vi "MultiStationGasMeter_Rev0.vi"() -> ()   [LabVIEW 2014]
uses:
  <vilib>/DAQmx/read.llb/DAQmx Read (Analog 1D DBL NChan 1Samp).vi
  <vilib>/DAQmx/miscellaneous.llb/DAQmx Fill In Error Info.vi
panel:
  in  "HeatingValueLP 3":dbl=990.0 min=900.0 max=2600.0 step=1.0
  in  "HeatingValueNG 3":dbl=990.0 min=900.0 max=1200.0 step=1.0
  in  "Start ANSI 3":bool
  out "ANSI Average (BTU/hr) 3":dbl format="%#_5g"
  out "30 Second Average (BTU/hr) 3":dbl format="%#_5g"
  out "15 Second Average (BTU/hr) 3":dbl format="%#_5g"
  out "Signal 3":bool
  out "CF/HR 3":dbl format="%#_2g"
  out "HV 3":dbl
  out "Meter ID 3":dbl
  out "Gas 3":string
  out "DisplayChart 3":cluster{"Flow Rate":dbl}(graph)
  out "Flow Rate 3":dbl format="%#_5g"
  in  "HeatingValueLP 2":dbl=990.0 min=900.0 max=2600.0 step=1.0
  in  "Start ANSI 2":bool
  out "ANSI Average (BTU/hr) 2":dbl format="%#_5g"
  out "30 Second Average (BTU/hr) 2":dbl format="%#_5g"
  out "15 Second Average (BTU/hr) 2":dbl format="%#_5g"
  out "Signal 2":bool
  out "CF/HR 2":dbl format="%#_2g"
  out "HV 2":dbl
  in  "HeatingValueNG 2":dbl=990.0 min=900.0 max=1200.0 step=1.0
  out "Meter ID 2":dbl
  out "Gas 2":string
  out "DisplayChart 2":cluster{"Flow Rate":dbl}(graph)
  out "Flow Rate 2":dbl format="%#_5g"
  out "ANSI Placeholder 3":dbl
  out "Start Time ANSI 3":dbl
  out "ANSI Placeholder 2":dbl
  out "Start Time ANSI 2":dbl
  out "Meter 6 Present":bool
  out "Meter 5 Present":bool
  out "Meter 4 Present":bool
  out "Meter 3 Present":bool
  out "Meter 2 Present":bool
  out "Meter 1 Present":bool
  out "Meter Type 6":string
  out "Meter Type 2":string
  out "Meter Type 4":string
  out "Meter Type 5":string
  out "Meter Type 3":string
  out "Meter Type 1":string
  out "Meter 6 Size":dbl
  out "Meter 5 Size":dbl
  out "Meter 4 Size":dbl
  out "Meter 3 Size":dbl
  out "Meter 2 Size":dbl
  out "Meter 1 Size":dbl
  out "ANSI Placeholder":dbl
  out "Start Time ANSI":dbl
  in  "Start ANSI":bool
  out "ANSI Average (BTU/hr)":dbl format="%#_5g"
  out "30 Second Average (BTU/hr)":dbl format="%#_5g"
  out "15 Second Average (BTU/hr)":dbl format="%#_5g"
  out "Reference6":dbl
  out "Reference5":dbl
  out "Reference4":dbl
  out "Reference3":dbl
  out "Reference2":dbl
  out "Reference1":dbl
  out "Time":dbl
  out "Num Record":dbl
  in  "HeatingValueLP":dbl=2450.0 min=2400.0 max=2600.0 step=1.0
  out "Output 6":dbl min=0.0 max=5.0 step=0.01
  out "Output 5":dbl min=0.0 max=5.0 step=0.01
  out "Output 4":dbl min=0.0 max=5.0 step=0.01
  out "Output 3":dbl min=0.0 max=5.0 step=0.01
  out "Output 2":dbl min=0.0 max=5.0 step=0.01
  out "Output 1":dbl min=0.0 max=5.0 step=0.01
  out "Signal":bool
  in  "Record":bool
  out "File Path":path
  out "CF/HR":dbl format="%#_2g"
  out "HV":dbl
  in  "HeatingValueNG":dbl=990.0 min=900.0 max=1200.0 step=1.0
  out "Meter ID":dbl
  out "Gas":string
  out "DisplayChart":cluster{"Flow Rate":dbl}(graph)
  out "Flow Rate":dbl format="%#_5g"
  # "STATION 1"
  # "STATION 2"
  # "STATION 3"
  # "Heating Value"
  # "Heating Value"
  # "Heating Value"
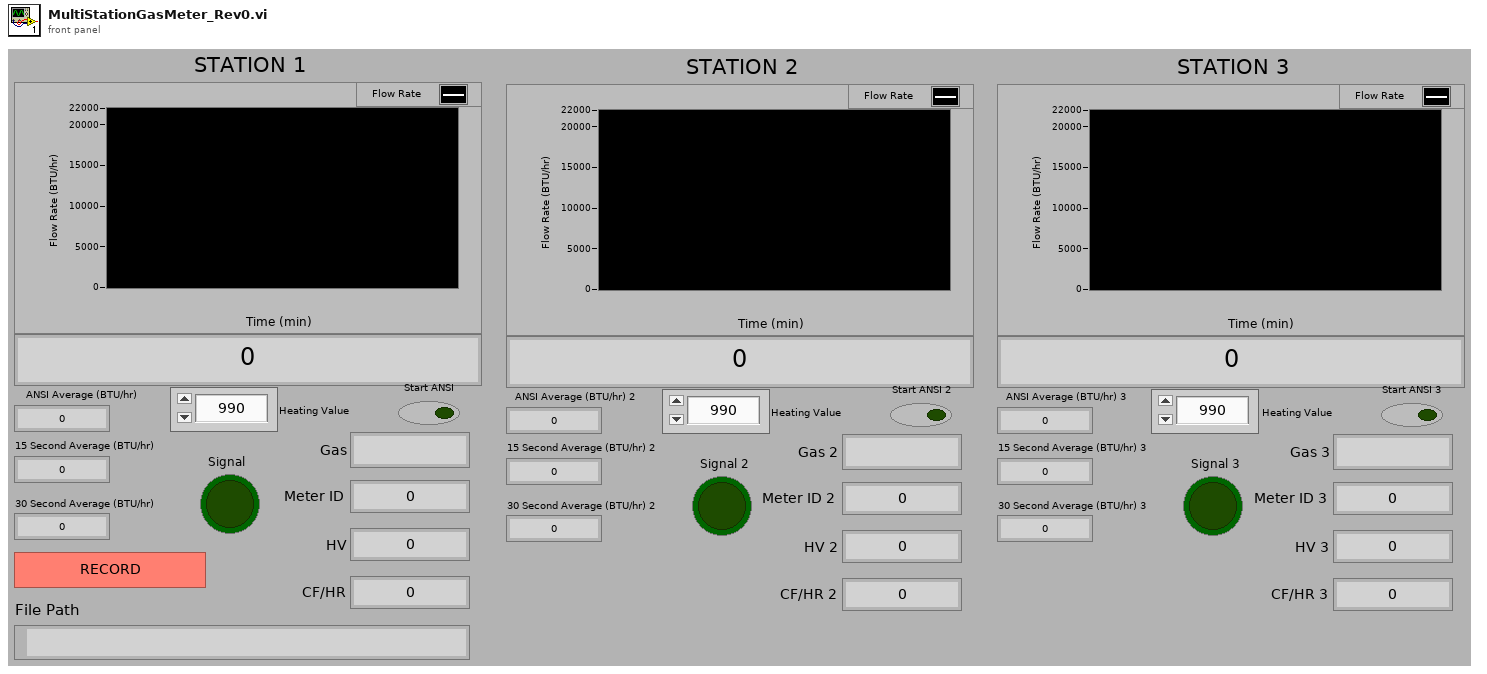
[diagram p1: front panel]
types:
  T1 = enum16{"open", "replace", "create", "open or create", "replace or create", "replace or create with confirmation"}
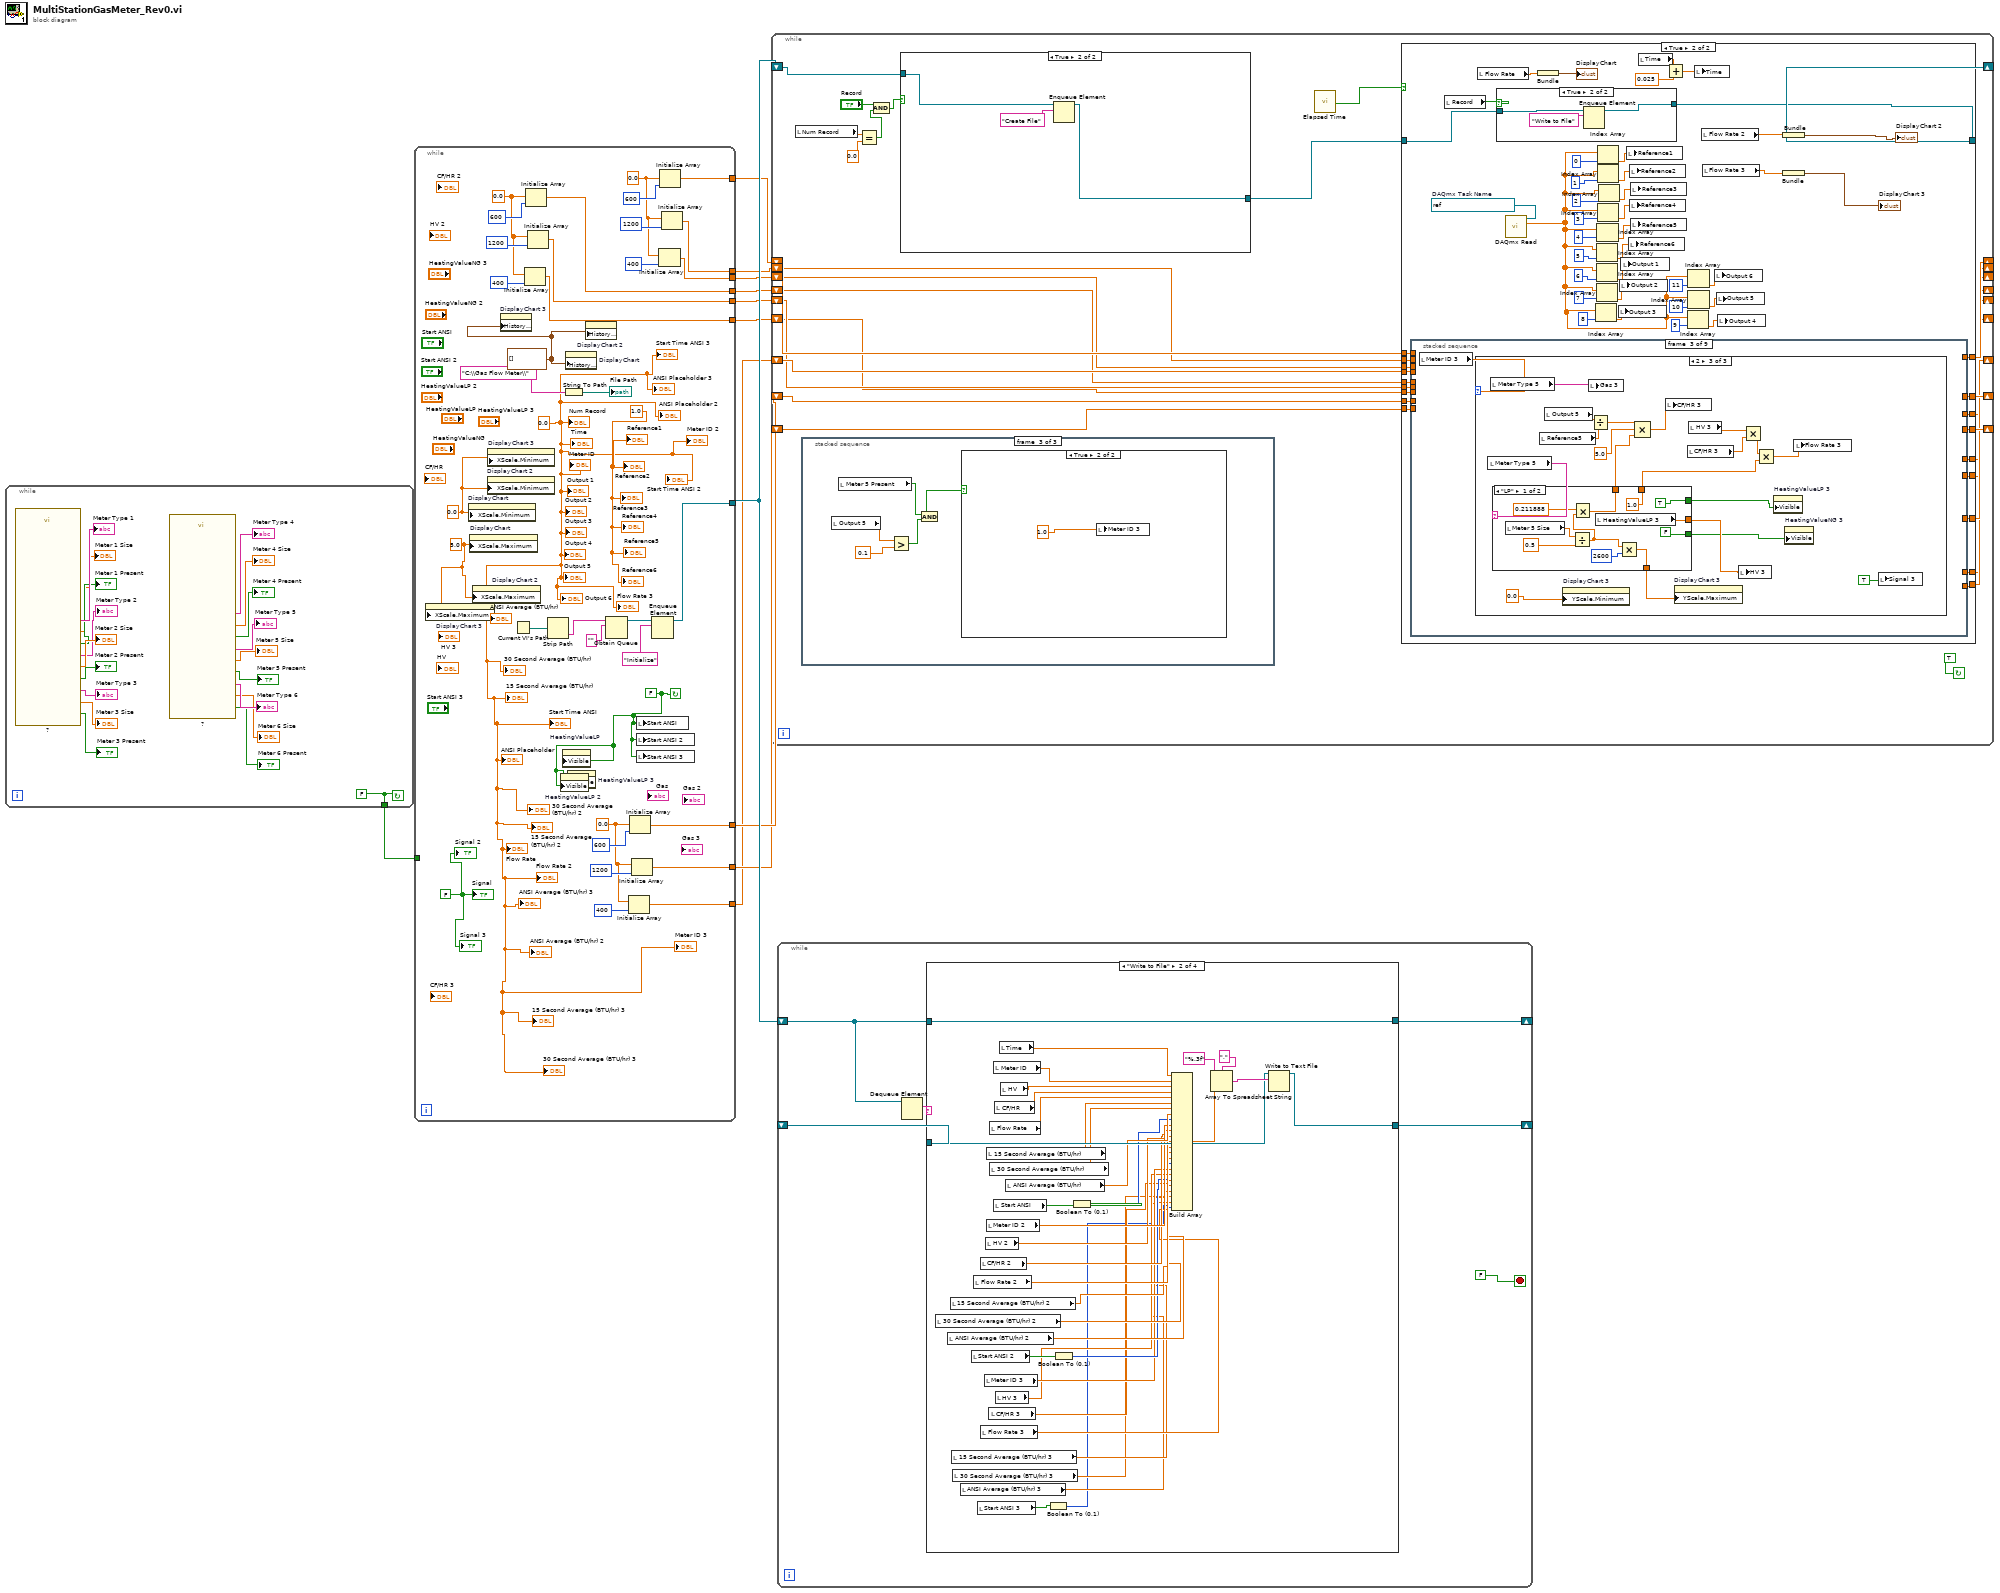
[diagram p0: block diagram]
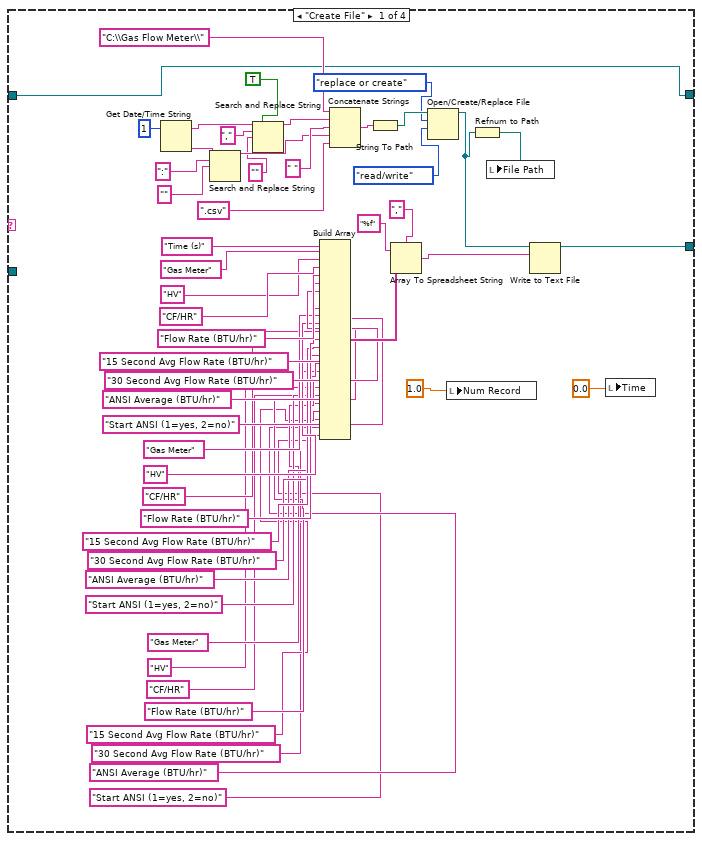
[diagram p2: hidden frame]
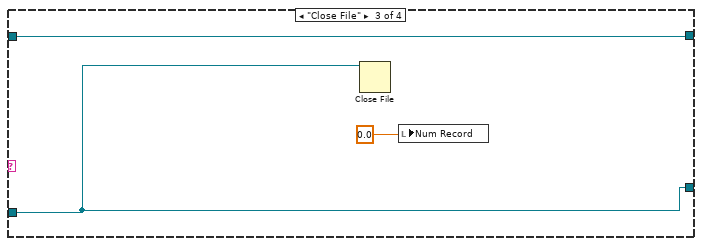
[diagram p3: hidden frame]
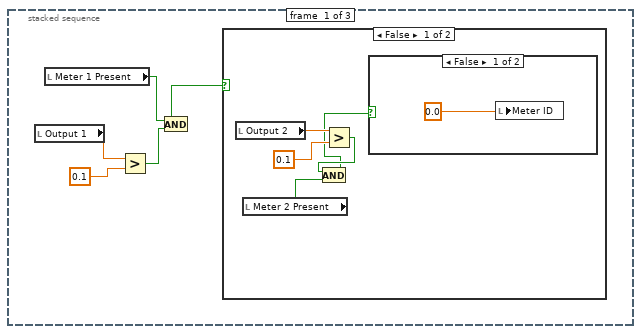
[diagram p5: hidden frame]
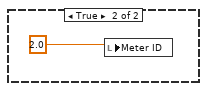
[diagram p6: hidden frame]
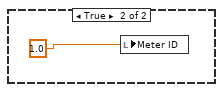
[diagram p7: hidden frame]
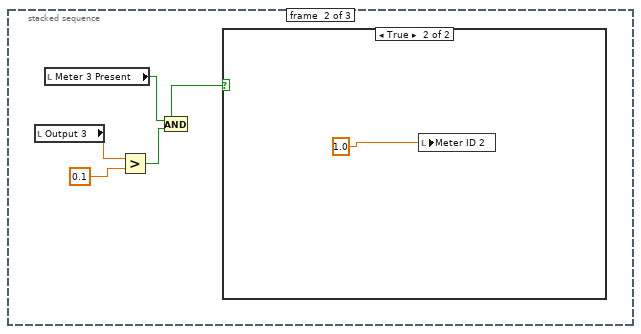
[diagram p8: hidden frame]
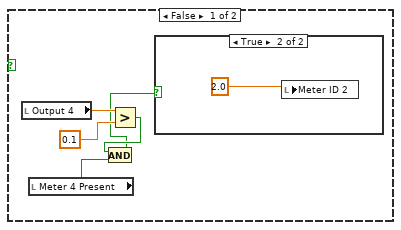
[diagram p9: hidden frame]
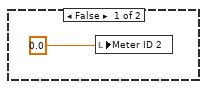
[diagram p10: hidden frame]
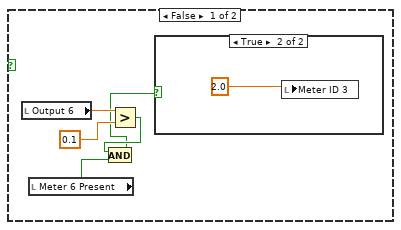
[diagram p11: hidden frame]
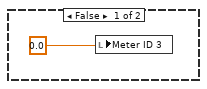
[diagram p12: hidden frame]
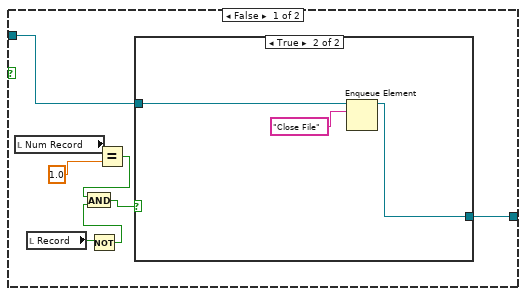
[diagram p13: hidden frame]
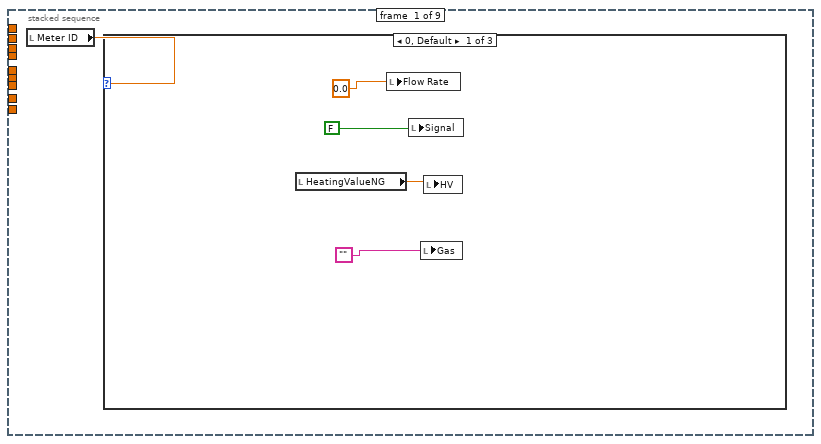
[diagram p16: hidden frame]
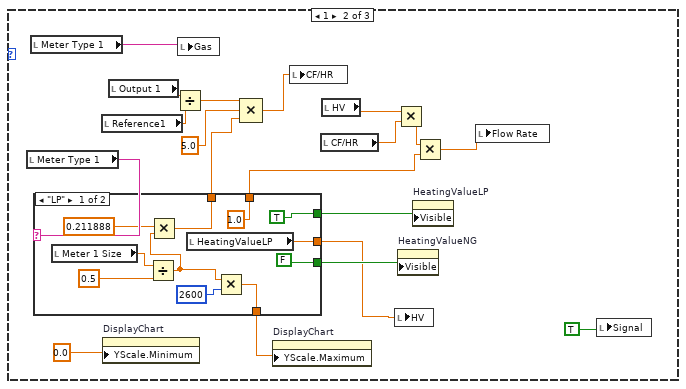
[diagram p17: hidden frame]
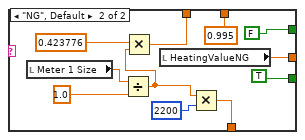
[diagram p18: hidden frame]
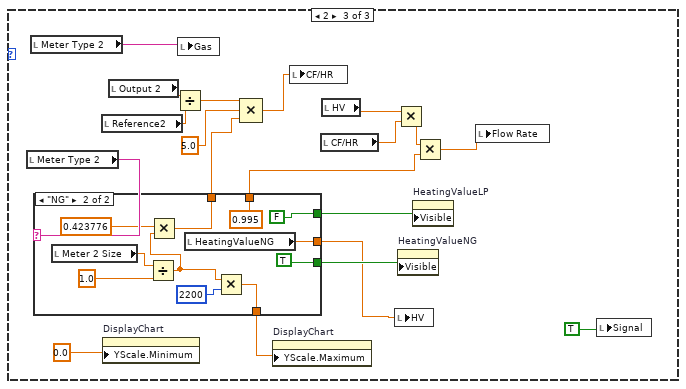
[diagram p19: hidden frame]
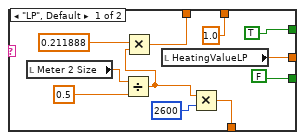
[diagram p20: hidden frame]
diagram:
  n1 = while {
    tunnel: [w29] -> w7
    stop <- w29 continue-if-true
    w29 = FALSE
    n2 = call "?"() -> ("Meter 3 Present?"=→"Meter 3 Present":bool, "Meter Size 3 (SLPM)"=→"Meter 3 Size":dbl, "Meter Type 3 (LP/NG)"=→"Meter Type 3":string, "Meter 2 Present?"=→"Meter 2 Present":bool, "Meter Size 2 (SLPM)"=→"Meter 2 Size":dbl, "Meter Type 2 (LP/NG)"=→"Meter Type 2":string, "Meter 1 Present?"=→"Meter 1 Present":bool, "Meter Size 1 (SLPM)"=→"Meter 1 Size":dbl, "Meter Type 1 (LP/NG)"=→"Meter Type 1":string)  [unwired: 9 in, 2 out]
    n3 = call "?"() -> ("Meter 6 Present?"=→"Meter 6 Present":bool, "Meter Size 6 (SLPM)"=→"Meter 6 Size":dbl, "Meter Type 6 (LP/NG)"=→"Meter Type 6":string, "Meter 5 Present?"=→"Meter 5 Present":bool, "Meter Size 5 (SLPM)"=→"Meter 5 Size":dbl, "Meter Type 5 (LP/NG)"=→"Meter Type 5":string, "Meter 4 Present?"=→"Meter 4 Present":bool, "Meter Size 4 (SLPM)"=→"Meter 4 Size":dbl, "Meter Type 4 (LP/NG)"=→"Meter Type 4":string)  [unwired: 9 in, 2 out]
  }
  n4 = while {
    tunnel: [w60] -> w11
    tunnel: [w56] -> w10
    tunnel: [w55] -> w9
    tunnel: [w52] -> w8
    tunnel: w7 -> [_]
    tunnel: [w47] -> w6
    tunnel: [w46] -> w5
    tunnel: [w45] -> w4
    tunnel: [w40] -> w3
    tunnel: [w39] -> w2
    tunnel: [w38] -> w1
    stop <- w36 continue-if-true
    w42 = 0.0
    w49 = 0.0
    w35 = FALSE
    w54 = 0.0
    w31 = 5.0
    w32 = 0.0
    w59 = 1.0
    w34 = 0.0
    w33 = cluster{"[0]":dbl}[] []
    w36 = FALSE
    n5 = property on="DisplayChart 3" class="WFChart (strict)"("XScale.Maximum"=w31) -> ()  [unwired: 2 in, 2 out]
    n6 = property on="DisplayChart" class="WFChart (strict)"("XScale.Minimum"=w32) -> ()  [unwired: 2 in, 2 out]
    n7 = property on="DisplayChart" class="WFChart (strict)"("XScale.Maximum"=w31) -> ()  [unwired: 2 in, 2 out]
    n8 = property on="DisplayChart 2" class="WFChart (strict)"("XScale.Maximum"=w31) -> ()  [unwired: 2 in, 2 out]
    n9 = property on="DisplayChart 2" class="WFChart (strict)"("XScale.Minimum"=w32) -> ()  [unwired: 2 in, 2 out]
    n10 = property on="DisplayChart 3" class="WFChart (strict)"("XScale.Minimum"=w32) -> ()  [unwired: 2 in, 2 out]
    n11 = property on="DisplayChart 3" class="WFChart (strict)"("History Data"=w33) -> ()  [unwired: 2 in, 2 out]
    n12 = Current VI's Path() -> (path=w65:path)
    n13 = Initialize Array(w42, 400) -> (w38:dbl[])
    n14 = Initialize Array(w42, 600) -> (w40:dbl[])
    n15 = Initialize Array(w42, 1200) -> (w39:dbl[])
    n16 = Strip Path(path=w65) -> (name=w63:string)  [unwired: 1 out]
    n17 = property on="HeatingValueLP 2" class="DigNum (strict)"("Visible"=w36) -> ()  [unwired: 2 in, 2 out]
    n18 = property on="HeatingValueLP" class="DigNum (strict)"("Visible"=w36) -> ()  [unwired: 2 in, 2 out]
    n19 = String To Path(string="C:\\Gas Flow Meter\\") -> (path=→"File Path":path)
    n20 = property on="DisplayChart" class="WFChart (strict)"("History Data"=w33) -> ()  [unwired: 2 in, 2 out]
    n21 = property on="HeatingValueLP 3" class="DigNum (strict)"("Visible"=w36) -> ()  [unwired: 2 in, 2 out]
    n22 = property on="DisplayChart 2" class="WFChart (strict)"("History Data"=w33) -> ()  [unwired: 2 in, 2 out]
    n23 = Obtain Queue(name (unnamed)=w63, element data type="") -> (queue out=w61:refnum<queue>)  [unwired: 3 in, 2 out]
    n24 = Initialize Array(w54, 400) -> (w52:dbl[])
    n25 = Initialize Array(w54, 600) -> (w56:dbl[])
    n26 = Initialize Array(w54, 1200) -> (w55:dbl[])
    n27 = local write "Start ANSI"(w36) -> ()
    n28 = local write "Start ANSI 2"(w36) -> ()
    n29 = local write "Start ANSI 3"(w36) -> ()
    n30 = Enqueue Element(queue=w61, element="Initialize") -> (queue out=w60:refnum<queue>)  [unwired: 2 in, 2 out]
    n31 = Initialize Array(w49, 400) -> (w45:dbl[])
    n32 = Initialize Array(w49, 600) -> (w47:dbl[])
    n33 = Initialize Array(w49, 1200) -> (w46:dbl[])
    "Num Record" <- w34
    "Time" <- w34
    "Meter ID" <- w34
    "Output 1" <- w34
    "Output 2" <- w34
    "Output 3" <- w34
    "Output 4" <- w34
    "Output 5" <- w34
    "Output 6" <- w34
    "Reference1" <- w59
    "Reference2" <- w59
    "Reference3" <- w59
    "Reference4" <- w59
    "Reference5" <- w59
    "Reference6" <- w59
    "30 Second Average (BTU/hr)" <- w34
    "15 Second Average (BTU/hr)" <- w34
    "ANSI Average (BTU/hr)" <- w34
    "Start Time ANSI" <- w34
    "ANSI Placeholder" <- w34
    "Flow Rate" <- w34
    "Signal" <- w35
    "Start Time ANSI 3" <- w34
    "ANSI Placeholder 3" <- w34
    "ANSI Placeholder 2" <- w34
    "Start Time ANSI 2" <- w34
    "Signal 2" <- w35
    "Flow Rate 2" <- w34
    "ANSI Average (BTU/hr) 2" <- w34
    "Meter ID 2" <- w34
    "30 Second Average (BTU/hr) 2" <- w34
    "15 Second Average (BTU/hr) 2" <- w34
    "Signal 3" <- w35
    "Flow Rate 3" <- w34
    "Meter ID 3" <- w34
    "ANSI Average (BTU/hr) 3" <- w34
    "15 Second Average (BTU/hr) 3" <- w34
    "30 Second Average (BTU/hr) 3" <- w34
  }
  n34 = while {
    shift-right: [w92] -> _
    shift-left: w11 -> [w85]
    shift-right: [w91] -> _
    shift-left: w10 -> [w89]
    shift-right: [w90] -> _
    shift-left: w9 -> [w88]
    shift-right: [w87] -> _
    shift-left: w8 -> [w86]
    shift-right: [w77] -> _
    shift-left: w6 -> [w78]
    shift-right: [w75] -> _
    shift-left: w5 -> [w76]
    shift-right: [w73] -> _
    shift-left: w4 -> [w74]
    shift-right: [w71] -> _
    shift-left: w3 -> [w72]
    shift-right: [w69] -> _
    shift-left: w2 -> [w70]
    shift-right: [w67] -> _
    shift-left: w1 -> [w68]
    stop <- TRUE continue-if-true
    n35 = local read "Num Record"() -> (w81:dbl)
    n36 = stacked-sequence {
      frame #0 {
        n37 = local read "Output 1"() -> (w99:dbl)
        n38 = local read "Meter 1 Present"() -> (w96:bool)
        n39 = Greater?(x=w99, y=0.1) -> (0:w97:bool)
        n40 = And(x=w96, y=w97) -> (x .and. y?=w95:bool)
        n41 = case shown="False" w95 {
          frame False {
            n42 = local read "Output 2"() -> (w103:dbl)
            n43 = local read "Meter 2 Present"() -> (w102:bool)
            n44 = Greater?(x=w103, y=0.1) -> (0:w101:bool)
            n45 = And(x=w101, y=w102) -> (x .and. y?=w100:bool)
            n46 = case shown="False" w100 {
              frame False {
                n47 = local write "Meter ID"(0.0) -> ()
              }
              frame True {
                n48 = local write "Meter ID"(2.0) -> ()
              }
            }
          }
          frame True {
            n49 = local write "Meter ID"(1.0) -> ()
          }
        }
      }
      frame #1 {
        n50 = local read "Output 3"() -> (w112:dbl)
        n51 = local read "Meter 3 Present"() -> (w109:bool)
        n52 = Greater?(x=w112, y=0.1) -> (0:w110:bool)
        n53 = And(x=w109, y=w110) -> (x .and. y?=w108:bool)
        n54 = case shown="True" w108 {
          frame False {
            n55 = local read "Output 4"() -> (w116:dbl)
            n56 = local read "Meter 4 Present"() -> (w115:bool)
            n57 = Greater?(x=w116, y=0.1) -> (0:w114:bool)
            n58 = And(x=w114, y=w115) -> (x .and. y?=w113:bool)
            n59 = case shown="True" w113 {
              frame False {
                n60 = local write "Meter ID 2"(0.0) -> ()
              }
              frame True {
                n61 = local write "Meter ID 2"(2.0) -> ()
              }
            }
          }
          frame True {
            n62 = local write "Meter ID 2"(1.0) -> ()
          }
        }
      }
      frame #2 {
        n63 = local read "Output 5"() -> (w125:dbl)
        n64 = local read "Meter 5 Present"() -> (w122:bool)
        n65 = Greater?(x=w125, y=0.1) -> (0:w123:bool)
        n66 = And(x=w122, y=w123) -> (x .and. y?=w121:bool)
        n67 = case shown="True" w121 {
          frame False {
            n68 = local read "Output 6"() -> (w129:dbl)
            n69 = local read "Meter 6 Present"() -> (w128:bool)
            n70 = Greater?(x=w129, y=0.1) -> (0:w127:bool)
            n71 = And(x=w127, y=w128) -> (x .and. y?=w126:bool)
            n72 = case shown="True" w126 {
              frame False {
                n73 = local write "Meter ID 3"(0.0) -> ()
              }
              frame True {
                n74 = local write "Meter ID 3"(2.0) -> ()
              }
            }
          }
          frame True {
            n75 = local write "Meter ID 3"(1.0) -> ()
          }
        }
      }
    }
    n76 = Equal?(x=w81, y=0.0) -> (x = y?=w80:bool)
    n77 = And(x="Record", y=w80) -> (x .and. y?=w79:bool)
    n78 = case shown="True" w79 {
      tunnel: w85 -> [w139 w147]
      tunnel: [w138 w146] -> w84
      frame False {
        n79 = local read "Num Record"() -> (w141:dbl)
        n80 = local read "Record"() -> (w135:bool)
        n81 = Not(x=w135) -> (.not. x?=w134:bool)
        n82 = Equal?(x=w141, y=1.0) -> (x = y?=w137:bool)
        n83 = And(x=w137, y=w134) -> (x .and. y?=w136:bool)
        n84 = case shown="True" w136 {
          tunnel: w139 -> [w142 w144]
          tunnel: [w142 w143] -> w138
          frame False {
          }
          frame True {
            n85 = Enqueue Element(queue=w144, element="Close File") -> (queue out=w143:refnum<queue>)  [unwired: 2 in, 2 out]
          }
        }
      }
      frame True {
        n86 = Enqueue Element(queue=w147, element="Create File") -> (queue out=w146:refnum<queue>)  [unwired: 2 in, 2 out]
      }
    }
    n87 = call "Elapsed Time"() -> ("Time has Elapsed"=w93:bool)  [unwired: 12 in, 7 out]
    n88 = case shown="True" w93 {
      tunnel: w84 -> [w158 w208]
      tunnel: [w158 w207] -> w92
      tunnel: w89 -> [w157 w180]
      tunnel: w88 -> [w156 w179]
      tunnel: [w157 w178] -> w91
      tunnel: [w156 w177] -> w90
      tunnel: w86 -> [w155 w176]
      tunnel: [w155 w175] -> w87
      tunnel: w78 -> [w152 w174]
      tunnel: [w152 w173] -> w77
      tunnel: w76 -> [w153 w172]
      tunnel: [w153 w171] -> w75
      tunnel: w74 -> [w154 w170]
      tunnel: [w154 w169] -> w73
      tunnel: w72 -> [w151 w168]
      tunnel: [w151 w167] -> w71
      tunnel: w70 -> [w150 w166]
      tunnel: [w150 w165] -> w69
      tunnel: w68 -> [w149 w164]
      tunnel: [w149 w163] -> w67
      frame False {
      }
      frame True {
        w206 = refnum<k21> "ReadFlowMeterIn"  # DAQmx Task Name
        n89 = stacked-sequence {
          tunnel: w180 -> [_ _ _ w500 _ _ _ _ _]
          tunnel: w179 -> [_ _ _ w499 _ _ _ _ _]
          tunnel: [_ _ _ w494 _ _ _ _ _] -> w178
          tunnel: [_ _ _ w490 _ _ _ _ _] -> w177
          tunnel: w176 -> [_ _ _ w484 _ _ _ _ _]
          tunnel: [_ _ _ w481 _ _ _ _ _] -> w175
          tunnel: w174 -> [_ _ _ _ w523 _ _ _ _]
          tunnel: [_ _ _ _ w510 _ _ _ _] -> w173
          tunnel: w172 -> [_ _ _ _ w517 _ _ _ _]
          tunnel: [_ _ _ _ w509 _ _ _ _] -> w171
          tunnel: w170 -> [_ _ _ _ w515 _ _ _ _]
          tunnel: [_ _ _ _ w508 _ _ _ _] -> w169
          tunnel: w168 -> [_ _ _ _ _ w544 _ _ _]
          tunnel: [_ _ _ _ _ w542 _ _ _] -> w167
          tunnel: w166 -> [_ _ _ _ _ w541 _ _ _]
          tunnel: [_ _ _ _ _ w539 _ _ _] -> w165
          tunnel: w164 -> [_ _ _ _ _ w538 _ _ _]
          tunnel: [_ _ _ _ _ w536 _ _ _] -> w163
          frame #0 {
            n90 = local read "Meter ID"() -> (w215:dbl)
            n91 = case shown="0, Default" w215 {
              frame 0, Default {
                n92 = local read "HeatingValueNG"() -> (w219:dbl)
                n93 = local write "Flow Rate"(0.0) -> ()
                n94 = local write "Signal"(FALSE) -> ()
                n95 = local write "Gas"("") -> ()
                n96 = local write "HV"(w219) -> ()
              }
              frame 1 {
                n97 = local read "Meter Type 1"() -> (w228:string)
                n98 = local read "Meter Type 1"() -> (w222:string)
                n99 = case shown="\"LP\"" w228 {
                  tunnel: [w246 w257] -> w227
                  tunnel: [TRUE FALSE] -> w226
                  tunnel: [FALSE TRUE] -> w225
                  tunnel: [1.0 0.995] -> w224
                  tunnel: [w240 w251] -> w223
                  tunnel: [w239 w250] -> w221
                  frame "LP" {
                    n100 = local read "Meter 1 Size"() -> (w248:dbl)
                    n101 = Divide(x=w248, y=0.5) -> (x/y=w241:dbl)
                    n102 = Multiply(x=0.211888, y=w241) -> (x*y=w246:dbl)
                    n103 = local read "HeatingValueLP"() -> (w239:dbl)
                    n104 = Multiply(x=w241, y=2600) -> (x*y=w240:dbl)
                  }
                  frame "NG", Default {
                    n105 = local read "Meter 1 Size"() -> (w259:dbl)
                    n106 = Divide(x=w259, y=1.0) -> (x/y=w252:dbl)
                    n107 = Multiply(x=0.423776, y=w252) -> (x*y=w257:dbl)
                    n108 = local read "HeatingValueNG"() -> (w250:dbl)
                    n109 = Multiply(x=w252, y=2200) -> (x*y=w251:dbl)
                  }
                }
                n110 = local read "Reference1"() -> (w232:dbl)
                n111 = property on="DisplayChart" class="WFChart (strict)"("YScale.Minimum"=0.0) -> ()  [unwired: 2 in, 2 out]
                n112 = local read "Output 1"() -> (w233:dbl)
                n113 = Divide(x=w233, y=w232) -> (x/y=w230:dbl)
                n114 = local write "Gas"(w222) -> ()
                n115 = Compound Arithmetic op=MULTIPLY(w230, 5.0, w227) -> (w220:dbl)
                n116 = property on="DisplayChart" class="WFChart (strict)"("YScale.Maximum"=w223) -> ()  [unwired: 2 in, 2 out]
                n117 = local write "CF/HR"(w220) -> ()
                n118 = local read "CF/HR"() -> (w235:dbl)
                n119 = local read "HV"() -> (w234:dbl)
                n120 = local write "HV"(w221) -> ()
                n121 = Multiply(x=w234, y=w235) -> (x*y=w236:dbl)
                n122 = property on="HeatingValueNG" class="DigNum (strict)"("Visible"=w225) -> ()  [unwired: 2 in, 2 out]
                n123 = property on="HeatingValueLP" class="DigNum (strict)"("Visible"=w226) -> ()  [unwired: 2 in, 2 out]
                n124 = Multiply(x=w236, y=w224) -> (x*y=w237:dbl)
                n125 = local write "Flow Rate"(w237) -> ()
                n126 = local write "Signal"(TRUE) -> ()
              }
              frame 2 {
                n127 = local read "Meter Type 2"() -> (w269:string)
                n128 = local read "Meter Type 2"() -> (w263:string)
                n129 = case shown="\"NG\"" w269 {
                  tunnel: [w287 w298] -> w268
                  tunnel: [TRUE FALSE] -> w267
                  tunnel: [FALSE TRUE] -> w266
                  tunnel: [1.0 0.995] -> w265
                  tunnel: [w281 w292] -> w264
                  tunnel: [w280 w291] -> w262
                  frame "LP", Default {
                    n130 = local read "Meter 2 Size"() -> (w289:dbl)
                    n131 = Divide(x=w289, y=0.5) -> (x/y=w282:dbl)
                    n132 = Multiply(x=0.211888, y=w282) -> (x*y=w287:dbl)
                    n133 = local read "HeatingValueLP"() -> (w280:dbl)
                    n134 = Multiply(x=w282, y=2600) -> (x*y=w281:dbl)
                  }
                  frame "NG" {
                    n135 = local read "Meter 2 Size"() -> (w300:dbl)
                    n136 = Divide(x=w300, y=1.0) -> (x/y=w293:dbl)
                    n137 = Multiply(x=0.423776, y=w293) -> (x*y=w298:dbl)
                    n138 = local read "HeatingValueNG"() -> (w291:dbl)
                    n139 = Multiply(x=w293, y=2200) -> (x*y=w292:dbl)
                  }
                }
                n140 = local read "Reference2"() -> (w273:dbl)
                n141 = property on="DisplayChart" class="WFChart (strict)"("YScale.Minimum"=0.0) -> ()  [unwired: 2 in, 2 out]
                n142 = local read "Output 2"() -> (w274:dbl)
                n143 = Divide(x=w274, y=w273) -> (x/y=w271:dbl)
                n144 = local write "Gas"(w263) -> ()
                n145 = Compound Arithmetic op=MULTIPLY(w271, 5.0, w268) -> (w261:dbl)
                n146 = property on="DisplayChart" class="WFChart (strict)"("YScale.Maximum"=w264) -> ()  [unwired: 2 in, 2 out]
                n147 = local write "CF/HR"(w261) -> ()
                n148 = local read "CF/HR"() -> (w276:dbl)
                n149 = local read "HV"() -> (w275:dbl)
                n150 = local write "HV"(w262) -> ()
                n151 = Multiply(x=w275, y=w276) -> (x*y=w277:dbl)
                n152 = property on="HeatingValueNG" class="DigNum (strict)"("Visible"=w266) -> ()  [unwired: 2 in, 2 out]
                n153 = property on="HeatingValueLP" class="DigNum (strict)"("Visible"=w267) -> ()  [unwired: 2 in, 2 out]
                n154 = Multiply(x=w277, y=w265) -> (x*y=w278:dbl)
                n155 = local write "Flow Rate"(w278) -> ()
                n156 = local write "Signal"(TRUE) -> ()
              }
            }
          }
          frame #1 {
            n157 = local read "Meter ID 2"() -> (w302:dbl)
            n158 = case shown="2" w302 {
              frame 0, Default {
                n159 = local read "HeatingValueNG 2"() -> (w306:dbl)
                n160 = local write "Flow Rate 2"(0.0) -> ()
                n161 = local write "Signal 2"(FALSE) -> ()
                n162 = local write "Gas 2"("") -> ()
                n163 = local write "HV 2"(w306) -> ()
              }
              frame 1 {
                n164 = local read "Meter Type 3"() -> (w316:string)
                n165 = local read "Meter Type 3"() -> (w313:string)
                n166 = case shown="\"LP\"" w316 {
                  tunnel: [w333 w344] -> w315
                  tunnel: [TRUE FALSE] -> w309
                  tunnel: [FALSE TRUE] -> w310
                  tunnel: [1.0 0.995] -> w314
                  tunnel: [w327 w338] -> w307
                  tunnel: [w326 w337] -> w312
                  frame "LP" {
                    n167 = local read "Meter 3 Size"() -> (w335:dbl)
                    n168 = Divide(x=w335, y=0.5) -> (x/y=w328:dbl)
                    n169 = Multiply(x=0.211888, y=w328) -> (x*y=w333:dbl)
                    n170 = local read "HeatingValueLP 2"() -> (w326:dbl)
                    n171 = Multiply(x=w328, y=2600) -> (x*y=w327:dbl)
                  }
                  frame "NG", Default {
                    n172 = local read "Meter 3 Size"() -> (w346:dbl)
                    n173 = Divide(x=w346, y=1.0) -> (x/y=w339:dbl)
                    n174 = Multiply(x=0.423776, y=w339) -> (x*y=w344:dbl)
                    n175 = local read "HeatingValueNG 2"() -> (w337:dbl)
                    n176 = Multiply(x=w339, y=2200) -> (x*y=w338:dbl)
                  }
                }
                n177 = local read "Reference3"() -> (w319:dbl)
                n178 = local read "Output 3"() -> (w320:dbl)
                n179 = property on="DisplayChart 2" class="WFChart (strict)"("YScale.Minimum"=0.0) -> ()  [unwired: 2 in, 2 out]
                n180 = local write "Gas 2"(w313) -> ()
                n181 = Divide(x=w320, y=w319) -> (x/y=w317:dbl)
                n182 = Compound Arithmetic op=MULTIPLY(w317, 5.0, w315) -> (w311:dbl)
                n183 = local write "CF/HR 2"(w311) -> ()
                n184 = property on="DisplayChart 2" class="WFChart (strict)"("YScale.Maximum"=w307) -> ()  [unwired: 2 in, 2 out]
                n185 = local read "CF/HR 2"() -> (w322:dbl)
                n186 = local read "HV 2"() -> (w321:dbl)
                n187 = local write "HV 2"(w312) -> ()
                n188 = Multiply(x=w321, y=w322) -> (x*y=w323:dbl)
                n189 = Multiply(x=w323, y=w314) -> (x*y=w324:dbl)
                n190 = property on="HeatingValueLP 2" class="DigNum (strict)"("Visible"=w309) -> ()  [unwired: 2 in, 2 out]
                n191 = property on="HeatingValueNG 2" class="DigNum (strict)"("Visible"=w310) -> ()  [unwired: 2 in, 2 out]
                n192 = local write "Flow Rate 2"(w324) -> ()
                n193 = local write "Signal 2"(TRUE) -> ()
              }
              frame 2 {
                n194 = local read "Meter Type 3"() -> (w357:string)
                n195 = local read "Meter Type 3"() -> (w354:string)
                n196 = case shown="\"LP\"" w357 {
                  tunnel: [w374 w385] -> w356
                  tunnel: [TRUE FALSE] -> w350
                  tunnel: [FALSE TRUE] -> w351
                  tunnel: [1.0 0.995] -> w355
                  tunnel: [w368 w379] -> w348
                  tunnel: [w367 w378] -> w353
                  frame "LP" {
                    n197 = local read "Meter 3 Size"() -> (w376:dbl)
                    n198 = Divide(x=w376, y=0.5) -> (x/y=w369:dbl)
                    n199 = Multiply(x=0.211888, y=w369) -> (x*y=w374:dbl)
                    n200 = local read "HeatingValueLP 2"() -> (w367:dbl)
                    n201 = Multiply(x=w369, y=2600) -> (x*y=w368:dbl)
                  }
                  frame "NG", Default {
                    n202 = local read "Meter 3 Size"() -> (w387:dbl)
                    n203 = Divide(x=w387, y=1.0) -> (x/y=w380:dbl)
                    n204 = Multiply(x=0.423776, y=w380) -> (x*y=w385:dbl)
                    n205 = local read "HeatingValueNG 2"() -> (w378:dbl)
                    n206 = Multiply(x=w380, y=2200) -> (x*y=w379:dbl)
                  }
                }
                n207 = local read "Reference3"() -> (w360:dbl)
                n208 = local read "Output 3"() -> (w361:dbl)
                n209 = property on="DisplayChart 2" class="WFChart (strict)"("YScale.Minimum"=0.0) -> ()  [unwired: 2 in, 2 out]
                n210 = local write "Gas 2"(w354) -> ()
                n211 = Divide(x=w361, y=w360) -> (x/y=w358:dbl)
                n212 = Compound Arithmetic op=MULTIPLY(w358, 5.0, w356) -> (w352:dbl)
                n213 = local write "CF/HR 2"(w352) -> ()
                n214 = property on="DisplayChart 2" class="WFChart (strict)"("YScale.Maximum"=w348) -> ()  [unwired: 2 in, 2 out]
                n215 = local read "CF/HR 2"() -> (w363:dbl)
                n216 = local read "HV 2"() -> (w362:dbl)
                n217 = local write "HV 2"(w353) -> ()
                n218 = Multiply(x=w362, y=w363) -> (x*y=w364:dbl)
                n219 = Multiply(x=w364, y=w355) -> (x*y=w365:dbl)
                n220 = property on="HeatingValueLP 2" class="DigNum (strict)"("Visible"=w350) -> ()  [unwired: 2 in, 2 out]
                n221 = property on="HeatingValueNG 2" class="DigNum (strict)"("Visible"=w351) -> ()  [unwired: 2 in, 2 out]
                n222 = local write "Flow Rate 2"(w365) -> ()
                n223 = local write "Signal 2"(TRUE) -> ()
              }
            }
          }
          frame #2 {
            n224 = local read "Meter ID 3"() -> (w389:dbl)
            n225 = case shown="2" w389 {
              frame 0, Default {
                n226 = local read "HeatingValueNG 3"() -> (w393:dbl)
                n227 = local write "Flow Rate 3"(0.0) -> ()
                n228 = local write "Signal 3"(FALSE) -> ()
                n229 = local write "Gas 3"("") -> ()
                n230 = local write "HV 3"(w393) -> ()
              }
              frame 1 {
                n231 = local read "Meter Type 5"() -> (w403:string)
                n232 = local read "Meter Type 5"() -> (w400:string)
                n233 = case shown="\"LP\"" w403 {
                  tunnel: [w420 w431] -> w402
                  tunnel: [TRUE FALSE] -> w396
                  tunnel: [FALSE TRUE] -> w397
                  tunnel: [1.0 0.995] -> w401
                  tunnel: [w414 w425] -> w395
                  tunnel: [w413 w424] -> w399
                  frame "LP" {
                    n234 = local read "Meter 5 Size"() -> (w422:dbl)
                    n235 = Divide(x=w422, y=0.5) -> (x/y=w415:dbl)
                    n236 = Multiply(x=0.211888, y=w415) -> (x*y=w420:dbl)
                    n237 = local read "HeatingValueLP 3"() -> (w413:dbl)
                    n238 = Multiply(x=w415, y=2600) -> (x*y=w414:dbl)
                  }
                  frame "NG", Default {
                    n239 = local read "Meter 5 Size"() -> (w433:dbl)
                    n240 = Divide(x=w433, y=1.0) -> (x/y=w426:dbl)
                    n241 = Multiply(x=0.423776, y=w426) -> (x*y=w431:dbl)
                    n242 = local read "HeatingValueNG 3"() -> (w424:dbl)
                    n243 = Multiply(x=w426, y=2200) -> (x*y=w425:dbl)
                  }
                }
                n244 = local read "Reference5"() -> (w406:dbl)
                n245 = local read "Output 5"() -> (w407:dbl)
                n246 = property on="DisplayChart 3" class="WFChart (strict)"("YScale.Minimum"=0.0) -> ()  [unwired: 2 in, 2 out]
                n247 = local write "Gas 3"(w400) -> ()
                n248 = Divide(x=w407, y=w406) -> (x/y=w404:dbl)
                n249 = Compound Arithmetic op=MULTIPLY(w404, 5.0, w402) -> (w398:dbl)
                n250 = local write "CF/HR 3"(w398) -> ()
                n251 = property on="DisplayChart 3" class="WFChart (strict)"("YScale.Maximum"=w395) -> ()  [unwired: 2 in, 2 out]
                n252 = local read "CF/HR 3"() -> (w409:dbl)
                n253 = local read "HV 3"() -> (w408:dbl)
                n254 = local write "HV 3"(w399) -> ()
                n255 = Multiply(x=w408, y=w409) -> (x*y=w410:dbl)
                n256 = Multiply(x=w410, y=w401) -> (x*y=w411:dbl)
                n257 = property on="HeatingValueLP 3" class="DigNum (strict)"("Visible"=w396) -> ()  [unwired: 2 in, 2 out]
                n258 = property on="HeatingValueNG 3" class="DigNum (strict)"("Visible"=w397) -> ()  [unwired: 2 in, 2 out]
                n259 = local write "Flow Rate 3"(w411) -> ()
                n260 = local write "Signal 3"(TRUE) -> ()
              }
              frame 2 {
                n261 = local read "Meter Type 5"() -> (w444:string)
                n262 = local read "Meter Type 5"() -> (w441:string)
                n263 = case shown="\"LP\"" w444 {
                  tunnel: [w461 w472] -> w443
                  tunnel: [TRUE FALSE] -> w437
                  tunnel: [FALSE TRUE] -> w438
                  tunnel: [1.0 0.995] -> w442
                  tunnel: [w455 w466] -> w436
                  tunnel: [w454 w465] -> w440
                  frame "LP" {
                    n264 = local read "Meter 5 Size"() -> (w463:dbl)
                    n265 = Divide(x=w463, y=0.5) -> (x/y=w456:dbl)
                    n266 = Multiply(x=0.211888, y=w456) -> (x*y=w461:dbl)
                    n267 = local read "HeatingValueLP 3"() -> (w454:dbl)
                    n268 = Multiply(x=w456, y=2600) -> (x*y=w455:dbl)
                  }
                  frame "NG", Default {
                    n269 = local read "Meter 5 Size"() -> (w474:dbl)
                    n270 = Divide(x=w474, y=1.0) -> (x/y=w467:dbl)
                    n271 = Multiply(x=0.423776, y=w467) -> (x*y=w472:dbl)
                    n272 = local read "HeatingValueNG 3"() -> (w465:dbl)
                    n273 = Multiply(x=w467, y=2200) -> (x*y=w466:dbl)
                  }
                }
                n274 = local read "Reference5"() -> (w447:dbl)
                n275 = local read "Output 5"() -> (w448:dbl)
                n276 = property on="DisplayChart 3" class="WFChart (strict)"("YScale.Minimum"=0.0) -> ()  [unwired: 2 in, 2 out]
                n277 = local write "Gas 3"(w441) -> ()
                n278 = Divide(x=w448, y=w447) -> (x/y=w445:dbl)
                n279 = Compound Arithmetic op=MULTIPLY(w445, 5.0, w443) -> (w439:dbl)
                n280 = local write "CF/HR 3"(w439) -> ()
                n281 = property on="DisplayChart 3" class="WFChart (strict)"("YScale.Maximum"=w436) -> ()  [unwired: 2 in, 2 out]
                n282 = local read "CF/HR 3"() -> (w450:dbl)
                n283 = local read "HV 3"() -> (w449:dbl)
                n284 = local write "HV 3"(w440) -> ()
                n285 = Multiply(x=w449, y=w450) -> (x*y=w451:dbl)
                n286 = Multiply(x=w451, y=w442) -> (x*y=w452:dbl)
                n287 = property on="HeatingValueLP 3" class="DigNum (strict)"("Visible"=w437) -> ()  [unwired: 2 in, 2 out]
                n288 = property on="HeatingValueNG 3" class="DigNum (strict)"("Visible"=w438) -> ()  [unwired: 2 in, 2 out]
                n289 = local write "Flow Rate 3"(w452) -> ()
                n290 = local write "Signal 3"(TRUE) -> ()
              }
            }
          }
          frame #3 {
            n291 = Delete From Array(array=w500, index=599) -> (array with subset deleted=w495:dbl[])  [unwired: 1 in, 1 out]
            n292 = Delete From Array(array=w484, index=399) -> (array with subset deleted=w482:dbl[])  [unwired: 1 in, 1 out]
            n293 = Delete From Array(array=w499, index=1199) -> (array with subset deleted=w496:dbl[])  [unwired: 1 in, 1 out]
            n294 = local read "Flow Rate"() -> (w477:dbl)
            n295 = Insert Into Array(array=w482, index=0, new element=w477) -> (w481:dbl[])
            n296 = Insert Into Array(array=w495, index=0, new element=w477) -> (w494:dbl[])
            n297 = Insert Into Array(array=w496, index=0, new element=w477) -> (w490:dbl[])
            n298 = Add Array Elements(numeric array=w481) -> (sum=w480:dbl)
            n299 = Array Size(array=w481) -> (size(s)=w479:i32)
            n300 = Add Array Elements(numeric array=w490) -> (sum=w489:dbl)
            n301 = Array Size(array=w490) -> (size(s)=w488:i32)
            n302 = Add Array Elements(numeric array=w494) -> (sum=w492:dbl)
            n303 = Array Size(array=w494) -> (size(s)=w493:i32)
            n304 = Divide(x=w480, y=w479) -> (x/y=w478:dbl)
            n305 = Divide(x=w489, y=w488) -> (x/y=w487:dbl)
            n306 = Divide(x=w492, y=w493) -> (x/y=w491:dbl)
            n307 = local write "15 Second Average (BTU/hr)"(w491) -> ()
            n308 = local write "ANSI Placeholder"(w478) -> ()
            n309 = local write "30 Second Average (BTU/hr)"(w487) -> ()
          }
          frame #4 {
            n310 = Delete From Array(array=w517, index=1199) -> (array with subset deleted=w516:dbl[])  [unwired: 1 in, 1 out]
            n311 = Delete From Array(array=w523, index=599) -> (array with subset deleted=w522:dbl[])  [unwired: 1 in, 1 out]
            n312 = Delete From Array(array=w515, index=399) -> (array with subset deleted=w514:dbl[])  [unwired: 1 in, 1 out]
            n313 = local read "Flow Rate 2"() -> (w504:dbl)
            n314 = Insert Into Array(array=w516, index=0, new element=w504) -> (w509:dbl[])
            n315 = Insert Into Array(array=w522, index=0, new element=w504) -> (w510:dbl[])
            n316 = Insert Into Array(array=w514, index=0, new element=w504) -> (w508:dbl[])
            n317 = Add Array Elements(numeric array=w509) -> (sum=w520:dbl)
            n318 = Array Size(array=w509) -> (size(s)=w521:i32)
            n319 = Add Array Elements(numeric array=w510) -> (sum=w524:dbl)
            n320 = Array Size(array=w510) -> (size(s)=w525:i32)
            n321 = Add Array Elements(numeric array=w508) -> (sum=w518:dbl)
            n322 = Array Size(array=w508) -> (size(s)=w519:i32)
            n323 = Divide(x=w520, y=w521) -> (x/y=w503:dbl)
            n324 = Divide(x=w524, y=w525) -> (x/y=w502:dbl)
            n325 = Divide(x=w518, y=w519) -> (x/y=w501:dbl)
            n326 = local write "30 Second Average (BTU/hr) 2"(w503) -> ()
            n327 = local write "15 Second Average (BTU/hr) 2"(w502) -> ()
            n328 = local write "ANSI Placeholder 2"(w501) -> ()
          }
          frame #5 {
            n329 = local read "Flow Rate 3"() -> (w535:dbl)
            n330 = Delete From Array(array=w541, index=1199) -> (array with subset deleted=w540:dbl[])  [unwired: 1 in, 1 out]
            n331 = Delete From Array(array=w538, index=399) -> (array with subset deleted=w537:dbl[])  [unwired: 1 in, 1 out]
            n332 = Delete From Array(array=w544, index=599) -> (array with subset deleted=w543:dbl[])  [unwired: 1 in, 1 out]
            n333 = Insert Into Array(array=w540, index=0, new element=w535) -> (w539:dbl[])
            n334 = Insert Into Array(array=w537, index=0, new element=w535) -> (w536:dbl[])
            n335 = Insert Into Array(array=w543, index=0, new element=w535) -> (w542:dbl[])
            n336 = Add Array Elements(numeric array=w539) -> (sum=w547:dbl)
            n337 = Add Array Elements(numeric array=w536) -> (sum=w545:dbl)
            n338 = Add Array Elements(numeric array=w542) -> (sum=w549:dbl)
            n339 = Array Size(array=w539) -> (size(s)=w548:i32)
            n340 = Array Size(array=w536) -> (size(s)=w546:i32)
            n341 = Array Size(array=w542) -> (size(s)=w550:i32)
            n342 = Divide(x=w547, y=w548) -> (x/y=w533:dbl)
            n343 = Divide(x=w545, y=w546) -> (x/y=w532:dbl)
            n344 = Divide(x=w549, y=w550) -> (x/y=w534:dbl)
            n345 = local write "30 Second Average (BTU/hr) 3"(w533) -> ()
            n346 = local write "15 Second Average (BTU/hr) 3"(w534) -> ()
            n347 = local write "ANSI Placeholder 3"(w532) -> ()
          }
          frame #6 {
            n348 = local read "Start ANSI"() -> (w551:bool)
            n349 = case shown="True" w551 {
              frame False {
              }
              frame True {
                n350 = local read "Start Time ANSI"() -> (w553:dbl)
                n351 = Equal?(x=w553, y=0.0) -> (x = y?=w552:bool)
                n352 = case shown="True" w552 {
                  frame False {
                    n353 = local read "Start Time ANSI"() -> (w559:dbl)
                    n354 = local read "Time"() -> (w556:dbl)
                    n355 = Add(x=w559, y=310) -> (x+y=w557:dbl)
                    n356 = Less Or Equal?(x=w556, y=w557) -> (x <= y?=w555:bool)
                    n357 = case shown="False" w555 {
                      frame False {
                        n358 = local read "ANSI Placeholder"() -> (w561:dbl)
                        n359 = local write "Start Time ANSI"(0.0) -> ()
                        n360 = local write "Start ANSI"(FALSE) -> ()
                        n361 = local write "ANSI Average (BTU/hr)"(w561) -> ()
                      }
                      frame True {
                      }
                    }
                  }
                  frame True {
                    n362 = local read "Time"() -> (w564:dbl)
                    n363 = local write "ANSI Average (BTU/hr)"(0.0) -> ()
                    n364 = local write "Start Time ANSI"(w564) -> ()
                  }
                }
              }
            }
          }
          frame #7 {
            n365 = local read "Start ANSI 2"() -> (w565:bool)
            n366 = case shown="True" w565 {
              frame False {
              }
              frame True {
                n367 = local read "Start Time ANSI 2"() -> (w567:dbl)
                n368 = Equal?(x=w567, y=0.0) -> (x = y?=w566:bool)
                n369 = case shown="False" w566 {
                  frame False {
                    n370 = local read "Start Time ANSI 2"() -> (w573:dbl)
                    n371 = local read "Time"() -> (w570:dbl)
                    n372 = Add(x=w573, y=310) -> (x+y=w571:dbl)
                    n373 = Less Or Equal?(x=w570, y=w571) -> (x <= y?=w569:bool)
                    n374 = case shown="False" w569 {
                      frame False {
                        n375 = local read "ANSI Placeholder 2"() -> (w575:dbl)
                        n376 = local write "Start Time ANSI 2"(0.0) -> ()
                        n377 = local write "Start ANSI 2"(FALSE) -> ()
                        n378 = local write "ANSI Average (BTU/hr) 2"(w575) -> ()
                      }
                      frame True {
                      }
                    }
                  }
                  frame True {
                    n379 = local read "Time"() -> (w578:dbl)
                    n380 = local write "ANSI Average (BTU/hr) 2"(0.0) -> ()
                    n381 = local write "Start Time ANSI 2"(w578) -> ()
                  }
                }
              }
            }
          }
          frame #8 {
            n382 = local read "Start ANSI 3"() -> (w579:bool)
            n383 = case shown="True" w579 {
              frame False {
              }
              frame True {
                n384 = local read "Start Time ANSI 3"() -> (w581:dbl)
                n385 = Equal?(x=w581, y=0.0) -> (x = y?=w580:bool)
                n386 = case shown="False" w580 {
                  frame False {
                    n387 = local read "Start Time ANSI 3"() -> (w587:dbl)
                    n388 = local read "Time"() -> (w584:dbl)
                    n389 = Add(x=w587, y=310) -> (x+y=w585:dbl)
                    n390 = Less Or Equal?(x=w584, y=w585) -> (x <= y?=w583:bool)
                    n391 = case shown="False" w583 {
                      frame False {
                        n392 = local read "ANSI Placeholder 3"() -> (w589:dbl)
                        n393 = local write "Start Time ANSI 3"(0.0) -> ()
                        n394 = local write "Start ANSI 3"(FALSE) -> ()
                        n395 = local write "ANSI Average (BTU/hr) 3"(w589) -> ()
                      }
                      frame True {
                      }
                    }
                  }
                  frame True {
                    n396 = local read "Time"() -> (w592:dbl)
                    n397 = local write "ANSI Average (BTU/hr) 3"(0.0) -> ()
                    n398 = local write "Start Time ANSI 3"(w592) -> ()
                  }
                }
              }
            }
          }
        }
        n399 = local read "Record"() -> (w212:bool)
        n400 = local read "Flow Rate"() -> (w214:dbl)
        n401 = case shown="True" w212 {
          tunnel: w208 -> [w593 w595]
          tunnel: [w593 w594] -> w207
          frame False {
          }
          frame True {
            n402 = Enqueue Element(queue=w595, element="Write to File") -> (queue out=w594:refnum<queue>)  [unwired: 2 in, 2 out]
          }
        }
        n403 = call-poly <vilib>:"DAQmx Read.vi"("task/channels in"=w206) -> ("data"=w205:dbl[])  [unwired: 12 in, 2 out]
        n404 = Bundle("Flow Rate"=w214) -> (→"DisplayChart":cluster{"Flow Rate":dbl})  [unwired: 1 in]
        n405 = Index Array(array=w205, index=8) -> (element=w189:dbl)
        n406 = Index Array(array=w205, index=5) -> (element=w186:dbl)
        n407 = Index Array(array=w205, index=6) -> (element=w187:dbl)
        n408 = Index Array(array=w205, index=7) -> (element=w188:dbl)
        n409 = Index Array(array=w205, index=4) -> (element=w185:dbl)
        n410 = Index Array(array=w205, index=0) -> (element=w181:dbl)
        n411 = Index Array(array=w205, index=1) -> (element=w182:dbl)
        n412 = Index Array(array=w205, index=3) -> (element=w184:dbl)
        n413 = Index Array(array=w205, index=2) -> (element=w183:dbl)
        n414 = local write "Output 3"(w189) -> ()
        n415 = local write "Output 2"(w188) -> ()
        n416 = local write "Output 1"(w187) -> ()
        n417 = local write "Reference1"(w181) -> ()
        n418 = local write "Reference6"(w186) -> ()
        n419 = local write "Reference2"(w182) -> ()
        n420 = local write "Reference4"(w184) -> ()
        n421 = local write "Reference3"(w183) -> ()
        n422 = local write "Reference5"(w185) -> ()
        n423 = local read "Time"() -> (w210:dbl)
        n424 = Add(x=w210, y=0.025) -> (x+y=w209:dbl)
        n425 = Index Array(array=w205, index=9) -> (element=w190:dbl)
        n426 = Index Array(array=w205, index=11) -> (element=w192:dbl)
        n427 = Index Array(array=w205, index=10) -> (element=w191:dbl)
        n428 = local write "Time"(w209) -> ()
        n429 = local read "Flow Rate 2"() -> (w162:dbl)
        n430 = local read "Flow Rate 3"() -> (w161:dbl)
        n431 = local write "Output 6"(w192) -> ()
        n432 = local write "Output 5"(w191) -> ()
        n433 = local write "Output 4"(w190) -> ()
        n434 = Bundle("Flow Rate 2"=w162) -> (→"DisplayChart 2":cluster{"Flow Rate 2":dbl})  [unwired: 1 in]
        n435 = Bundle("Flow Rate 3"=w161) -> (→"DisplayChart 3":cluster{"Flow Rate 3":dbl})  [unwired: 1 in]
      }
    }
  }
  n436 = while {
    shift-right: [w600] -> _
    shift-left: w11 -> [w597]
    shift-right: [w599] -> _
    shift-left: _ -> [w598]
    stop <- FALSE stop-if-true
    n437 = Dequeue Element(queue=w597) -> (element=w601:string)  [unwired: 2 in, 3 out]
    n438 = case shown="\"Write to File\"" w601 {
      tunnel: [w624 w680 w691 w694] -> w600
      tunnel: w597 -> [w624 w680 w691 w694]
      tunnel: [w623 w678 w690 w693] -> w599
      tunnel: w598 -> [_ w679 w690 w693]
      frame "Create File" {
        n439 = Get Date/Time String(date format (0)=1) -> (date string=w629:string, time string=w626:string)  [unwired: 2 in]
        n440 = Search and Replace String(input string=w626, search string=":", replace string="") -> (result string=w635:string)  [unwired: 5 in, 3 out]
        n441 = Search and Replace String(replace all?=TRUE, input string=w629, search string=",", replace string="") -> (result string=w636:string)  [unwired: 4 in, 3 out]
        n442 = Build Array("Time (s)", "Gas Meter", "HV", "CF/HR", "Flow Rate (BTU/hr)", "15 Second Avg Flow Rate (BTU/hr)", "30 Second Avg Flow Rate (BTU/hr)", "ANSI Average (BTU/hr)", "Start ANSI (1=yes, 2=no)", "Gas Meter", "HV", "CF/HR", "Flow Rate (BTU/hr)", "15 Second Avg Flow Rate (BTU/hr)", "30 Second Avg Flow Rate (BTU/hr)", "ANSI Average (BTU/hr)", "Start ANSI (1=yes, 2=no)", "Gas Meter", "HV", "CF/HR", "Flow Rate (BTU/hr)", "15 Second Avg Flow Rate (BTU/hr)", "30 Second Avg Flow Rate (BTU/hr)", "ANSI Average (BTU/hr)", "Start ANSI (1=yes, 2=no)") -> (w646:string[])
        n443 = Concatenate Strings("C:\\Gas Flow Meter\\", w636, " ", w635, ".csv") -> (w632:string)
        n444 = String To Path(string=w632) -> (path=w652:path)
        n445 = Array To Spreadsheet String(delimiter (Tab)=",", array=w646, 3:"%f" ("format string")) -> (spreadsheet string=w647:string)
        n446 = Open/Create/Replace File(file path (use dialog)=w652, operation (0:open)=T1."replace or create", access (0:read/write)=enum16{"read/write", "read-only", "write-only"}."read/write") -> (refnum out=w654:refnum<file>)  [unwired: 3 in, 2 out]
        n447 = local write "Num Record"(1.0) -> ()
        n448 = Refnum to Path(1:w654) -> (0:w653:path)
        n449 = local write "File Path"(w653) -> ()
        n450 = Write to Text File(file (use dialog)=w654, text=w647) -> (refnum out=w623:refnum<file>)  [unwired: 2 in, 2 out]
        n451 = local write "Time"(0.0) -> ()
      }
      frame "Write to File" {
        n452 = local read "30 Second Average (BTU/hr) 2"() -> (w665:dbl)
        n453 = local read "ANSI Average (BTU/hr) 2"() -> (w664:dbl)
        n454 = local read "15 Second Average (BTU/hr) 2"() -> (w666:dbl)
        n455 = local read "15 Second Average (BTU/hr) 3"() -> (w658:dbl)
        n456 = local read "30 Second Average (BTU/hr) 3"() -> (w657:dbl)
        n457 = local read "ANSI Average (BTU/hr) 3"() -> (w656:dbl)
        n458 = local read "Start ANSI 2"() -> (w671:bool)
        n459 = local read "Flow Rate 2"() -> (w667:dbl)
        n460 = local read "Start ANSI 3"() -> (w672:bool)
        n461 = local read "CF/HR 2"() -> (w668:dbl)
        n462 = local read "Flow Rate 3"() -> (w659:dbl)
        n463 = local read "Meter ID 3"() -> (w662:dbl)
        n464 = local read "HV 2"() -> (w669:dbl)
        n465 = local read "Meter ID 2"() -> (w670:dbl)
        n466 = local read "15 Second Average (BTU/hr)"() -> (w676:dbl)
        n467 = local read "CF/HR 3"() -> (w660:dbl)
        n468 = local read "Flow Rate"() -> (w683:dbl)
        n469 = local read "30 Second Average (BTU/hr)"() -> (w677:dbl)
        n470 = local read "Meter ID"() -> (w686:dbl)
        n471 = local read "Start ANSI"() -> (w674:bool)
        n472 = local read "CF/HR"() -> (w684:dbl)
        n473 = local read "HV 3"() -> (w661:dbl)
        n474 = local read "Time"() -> (w687:dbl)
        n475 = local read "HV"() -> (w685:dbl)
        n476 = local read "ANSI Average (BTU/hr)"() -> (w675:dbl)
        n477 = Boolean To (0,1)(Boolean=w672) -> (0, 1=w655:i16)
        n478 = Boolean To (0,1)(Boolean=w671) -> (0, 1=w663:i16)
        n479 = Boolean To (0,1)(Boolean=w674) -> (0, 1=w673:i16)
        n480 = Build Array(w687, w686, w685, w684, w683, w676, w677, w675, w673, w670, w669, w668, w667, w666, w665, w664, w663, w662, w661, w660, w659, w658, w657, w656, w655) -> (w682:dbl[])
        n481 = Array To Spreadsheet String(delimiter (Tab)=",", array=w682, 3:"%.3f" ("format string")) -> (spreadsheet string=w681:string)
        n482 = Write to Text File(file (use dialog)=w679, text=w681) -> (refnum out=w678:refnum<file>)  [unwired: 2 in, 2 out]
      }
      frame "Close File" {
        n483 = Close File(refnum=w690) -> ()  [unwired: 1 in, 2 out]
        n484 = local write "Num Record"(0.0) -> ()
      }
      frame "Initialize", Default {
      }
    }
  }
